vi "FPTemp.vi"() -> ()   [LabVIEW 2010]
uses:
  <vilib>/FieldPoint/Polymorphic Read.llb/FP Read (Float Array -IO).vi
panel:
  out "values":dbl[](array[numeric])
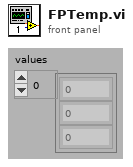
[diagram p1: front panel]
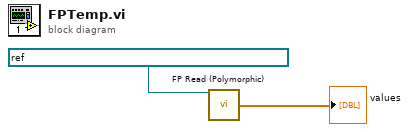
[diagram p0: block diagram]
diagram:
  n1 = call-poly <vilib>:"FP Read (Polymorphic).vi"("FieldPoint IO Point In"=refnum<k21> "FieldPoint\\FP @ COM1\\FP-TC-120 @11\\Ttem1 0") -> ("values"=→"values":dbl[])  [unwired: 11 in, 3 out]
